vi "Keithley2612b_NOT_Measurement_DC_Supply.vi"() -> ()   [LabVIEW 2016]
uses:
  <instrlib>/Keithley 2600 Series/Public/Channel.ctl
  <instrlib>/Keithley 2600 Series/Keithley 2600 Series.lvlib
  <instrlib>/BK Precision 913XX/BK Precision 913XX.lvlib
panel:
  in  "Appand to Exist File":bool
  in  "Write to Text File?":bool
  out "Actual Current Level (A)":dbl format="%.4g"
  out "Actual Power Level (W)":dbl format="%.4g"
  out "Actual Voltage Level (V)":dbl format="%.4g"
  out "XY Graph":cluster{"Y":dbl[], "Y":dbl[]}[](graph)=[{"Y"=[-10000.0, -9899.89, -9800.119999999999, -9699.970000000001, -9600.15, -9499.96, -9400.17, -9300.01, -9199.87, -9100.09, -8999.9, -8900.119999999999, -8800.0, -8700.18, -8600.02, -8499.88, -8400.080000000002, -8299.9, -8200.1, -8099.99, -8000.159999999999, -7899.9800000000005, -7799.92, -7700.11, -7599.95, -7500.15, -7400.0599999999995, -7300.21, -7200.05, -7099.96, -7000.14, -6900.0, -6800.21, -6700.08, -6599.910000000001, -6500.17, -6400.01, -6300.169999999999, -6200.0599999999995, -6100.25, -6000.110000000001, -5899.95, -5800.18, -5700.0599999999995, -5600.21, -5500.09, -5400.25, -5300.06, -5199.97, -5100.150000000001, -5000.0, -4900.2, -4800.03, -4700.21, -4600.06, -4499.93, -4400.13, -4299.98, -4200.160000000001, -4100.04, -4000.21, -3900.1299999999997, -3799.98, -3700.13, -3599.9900000000002, -3500.1600000000003, -3399.99, -3299.84, -3200.04, -3099.88, -3000.0499999999997, -2899.9, -2800.11, -2699.9300000000003, -2599.83, -2500.0, -2399.79, -2299.98, -2199.86, -2099.9900000000002, -1999.97, -1899.98, -1799.99, -1700.0, -1600.01, -1500.01, -1400.01, -1300.0100000000002, -1200.01, -1099.99, -999.993, -900.0, -800.006, -700.009, -600.01, -500.01399999999995, -400.01300000000003, -300.0, -199.989, -99.99470000000001, 0.00660419, 100.003, 200.002, 299.978, 399.99899999999997, 500.006, 600.0060000000001, 699.975, 799.9770000000001, 899.982, 999.977, 1099.98, 1199.9899999999998, 1300.0100000000002, 1399.97, 1499.98, 1599.99, 1699.9899999999998, 1799.98, 1899.97, 1999.96, 2099.75, 2199.91, 2299.77, 2399.88, 2499.76, 2599.9, 2699.71, 2799.88, 2900.04, 2999.85, 3100.04, 3199.84, 3300.02, 3399.81, 3500.0499999999997, 3599.8, 3699.9399999999996, 3800.11, 3899.96, 4000.0400000000004, 4099.95, 4200.0599999999995, 4299.87, 4400.070000000001, 4499.889999999999, 4600.030000000001, 4699.89, 4800.049999999999, 4900.1900000000005, 5000.0, 5100.150000000001, 5200.02, 5300.099999999999, 5399.969999999999, 5500.06, 5599.88, 5700.05, 5800.19, 5900.0, 6000.12, 6099.96, 6200.08, 6299.89, 6400.04, 6499.87, 6599.95, 6700.13, 6799.92, 6900.070000000001, 6999.91, 7099.99, 7199.82, 7299.9400000000005, 7399.82, 7499.94, 7600.1, 7699.92, 7800.07, 7899.84, 8000.04, 8099.84, 8199.91, 8299.810000000001, 8399.88, 8500.0, 8599.82, 8699.970000000001, 8799.73, 8899.88, 8999.75, 9099.949999999999, 9199.72, 9299.89, 9399.73, 9499.86, 9600.03, 9699.859999999999, 9800.01, 9899.84, 10000.0], "Y"=[4939.26, 4997.93, 4998.56, 4998.95, 4999.16, 4999.38, 4999.49, 4999.64, 4999.64, 4999.780000000001, 4999.83, 4999.87, 4999.88, 4999.95, 4999.92, 5000.0, 4999.98, 5000.02, 5000.05, 5000.06, 5000.09, 5000.09, 5000.08, 5000.13, 5000.15, 5000.15, 5000.200000000001, 5000.14, 5000.200000000001, 5000.17, 5000.2300000000005, 5000.200000000001, 5000.25, 5000.2300000000005, 5000.28, 5000.24, 5000.219999999999, 5000.27, 5000.27, 5000.19, 5000.27, 5000.21, 5000.29, 5000.25, 5000.27, 5000.28, 5000.29, 5000.27, 5000.3, 5000.25, 5000.339999999999, 5000.3099999999995, 5000.3, 5000.27, 5000.3, 5000.25, 5000.3099999999995, 5000.320000000001, 5000.3099999999995, 5000.3099999999995, 5000.3, 5000.320000000001, 5000.35, 5000.33, 5000.320000000001, 5000.33, 5000.3099999999995, 5000.320000000001, 5000.29, 5000.3099999999995, 5000.320000000001, 5000.33, 5000.35, 5000.339999999999, 5000.35, 5000.36, 5000.320000000001, 5000.36, 5000.35, 5000.35, 5000.35, 5000.36, 5000.320000000001, 5000.36, 5000.35, 5000.33, 5000.339999999999, 5000.320000000001, 5000.339999999999, 5000.33, 5000.339999999999, 5000.339999999999, 5000.36, 5000.339999999999, 5000.38, 5000.35, 5000.37, 5000.35, 5000.46, 5000.339999999999, 5000.41, 5000.36, 5000.39, 5000.37, 5000.429999999999, 5000.41, 5000.4, 5000.35, 5000.42, 5000.38, 5000.42, 5000.4400000000005, 5000.41, 5000.37, 5000.38, 5000.37, 5000.320000000001, 5000.38, 5000.39, 5000.39, 5000.38, 5000.42, 5000.37, 5000.4400000000005, 5000.36, 5000.37, 5000.41, 5000.39, 5000.41, 5000.42, 5000.37, 5000.39, 5000.36, 5000.4, 5000.41, 5000.42, 5000.339999999999, 5000.41, 5000.38, 5000.45, 5000.37, 5000.45, 5000.39, 5000.41, 5000.4, 5000.429999999999, 5000.38, 5000.42, 5000.38, 5000.4, 5000.41, 5000.42, 5000.42, 5000.37, 5000.4400000000005, 5000.39, 5000.429999999999, 5000.41, 5000.41, 5000.39, 5000.45, 5000.41, 5000.46, 5000.4, 5000.41, 5000.39, 5000.4400000000005, 5000.4, 5000.48, 5000.39, 5000.4, 5000.38, 5000.429999999999, 5000.45, 5000.4, 5000.41, 5000.4, 5000.42, 5000.42, 5000.429999999999, 5000.39, 5000.4400000000005, 5000.41, 5000.42, 5000.4, 5000.4400000000005, 5000.38, 5000.42, 5000.41, 5000.45, 5000.429999999999, 5000.48, 5000.49, 5000.47, 5000.5, 5000.429999999999, 5000.47, 5000.48, 5000.49, 5000.46, 5000.46]}]
  in  "Voltage Limit (36.000 V)":dbl=36.0 min=0.0 max=66.0 step=0.001 format="%.3g"
  in  "Enable OVP (T: Enable)":bool=TRUE
  in  "Channel (1:1)":u16(ring)=1 items=["1"=1, "2"=2, "3"=3]
  in  "Current Limit (0.0 A)":dbl=1.0 min=0.0 max=25.0 step=1.0 format="%.3f"
  in  "Voltage Level (0.0 V)":dbl=5.0 format="%.3g"
  in  "DC  VISA resource name":refnum<visa-resource-name>="bk_Precision_DC_Power"
  in  "Current Limit":dbl=1.0
  out "error out":errorcluster
  in  "DC Supply Delay (s)":dbl
  in  "Start Voltage 2":dbl=-10.0
  in  "Step Size":dbl=0.1
  in  "End Voltage":dbl=10.0
  in  "Delay (s)":dbl
  in  "Reverse Sweep":bool
  in  "error in (no error)":errorcluster
  in  "Keithley VISA resource name":refnum<visa-resource-name>="Keithley_2612B"
  # "DC Power Supply Control"
  # "Input Voltage Control"
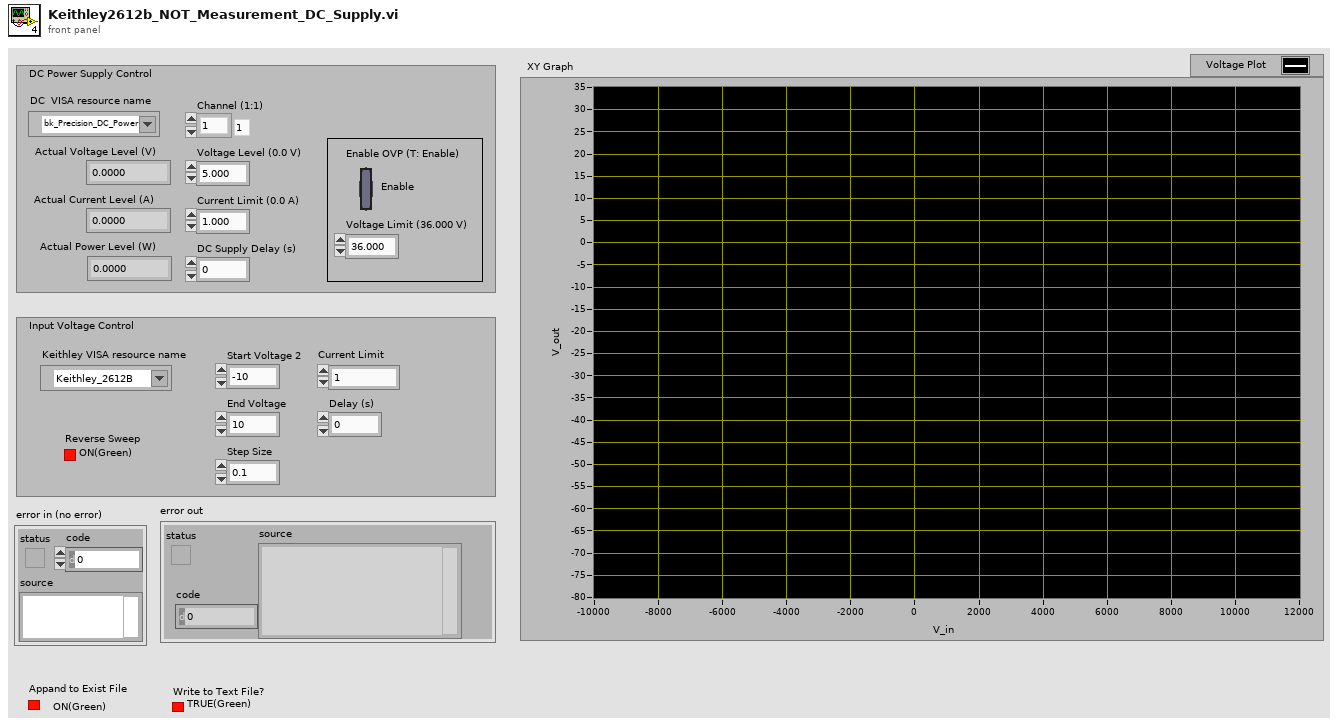
[diagram p1: front panel]
types:
  T1 = typedef "Keithley 2600 Series.lvlib/Channel.ctl" = enum32{"Channel A", "Channel B"}
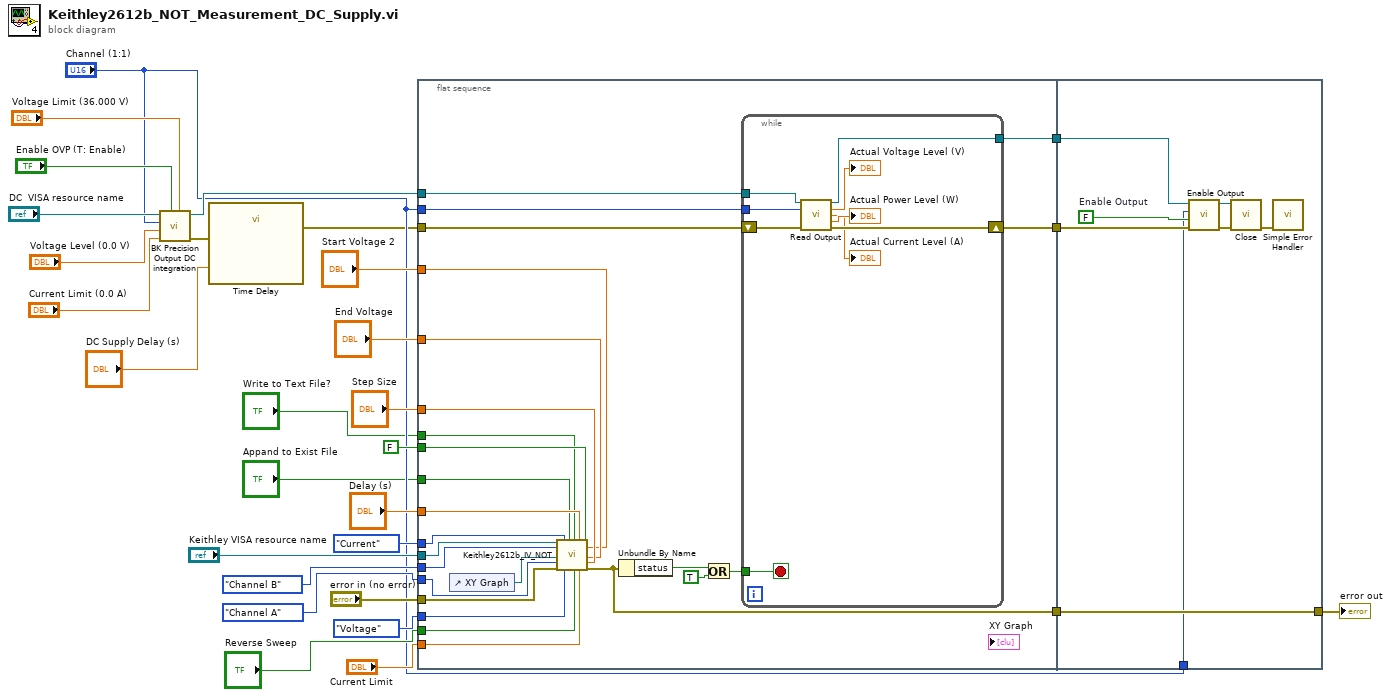
[diagram p0: block diagram]
diagram:
  n1 = call "BK Precision Output DC integration.vi"("Voltage Limit (36.000 V)"="Voltage Limit (36.000 V)", "Enable OVP (T: Enable)"="Enable OVP (T: Enable)", "Current Limit (0.0 A)"="Current Limit (0.0 A)", "Voltage Level (0.0 V)"="Voltage Level (0.0 V)", "Channel (1:1)"="Channel (1:1)", "VISA resource name"="DC  VISA resource name") -> ("error out"=w3:errorcluster, "VISA resource name out"=w7:refnum<visa-resource-name>)  [unwired: 2 in]
  n2 = call "Time Delay"("error in (no error)"=w3, "Delay Time (s)"="DC Supply Delay (s)") -> ("error out"=w4:errorcluster)  [unwired: 9 in]
  n3 = flat-sequence {
    tunnel: [w33] -> w15
    tunnel: "Current Limit" -> [w42]
    tunnel: "Start Voltage 2" -> [w43]
    tunnel: "Delay (s)" -> [w44]
    tunnel: "End Voltage" -> [w45]
    tunnel: "Step Size" -> [w46]
    tunnel: "Reverse Sweep" -> [w47]
    tunnel: enum32{"Current", "Voltage"}."Current" ("Source Function (Current)") -> [w48]
    tunnel: enum32{"Current", "Voltage"}."Voltage" ("Source Function (Current) 2") -> [w49]
    tunnel: Channel."Channel B" ("Channel (Channel A) 2") -> [w50]
    tunnel: Channel."Channel A" ("Channel (Channel A)") -> [w51]
    tunnel: "error in (no error)" -> [w52]
    tunnel: FALSE ("Error Query (False)") -> [w53]
    tunnel: "Keithley VISA resource name" -> [w54]
    tunnel: [w40] -> w8
    tunnel: w7 -> [w38]
    tunnel: [w39] -> w6
    tunnel: "Channel (1:1)" -> [w37]
    tunnel: w4 -> [w36]
    tunnel: "Appand to Exist File" -> [w31]
    tunnel: "Write to Text File?" -> [w30]
    tunnel: [w71] -> w17
    tunnel: w15 -> [w71]
    tunnel: w8 -> [w66]
    tunnel: "Channel (1:1)" -> [w64]
    tunnel: w6 -> [w65]
    frame #0 {
      n4 = control-ref of="XY Graph"() -> (w41:refnum<vi>)
      n5 = call "Keithley2612b_IV_NOT.vi"("VISA resource name"=w54, "Channel (Channel A) 2"=w50, "XY Graph Ref In"=w41, "Channel (Channel A)"=w51, "error in (no error)"=w52, "Source Function (Current)"=w48, "Source Function (Current) 2"=w49, "Appand to Exist File"=w31, "Write to Text File?"=w30, "Reverse Sweep"=w47, "Delay (s) 2"=w44, "Current Limit 2"=w42, "Error Query (False)"=w53, "Start Voltage 2"=w43, "End Voltage 2"=w45, "Step Size 2"=w46) -> ("error out"=w33:errorcluster)  [unwired: 3 in]
      n6 = Unbundle By Name(w33) -> ("status"=w34:bool)
      n7 = Or(x=w34, y=TRUE ("Stop Output")) -> (x .or. y?=w32:bool)
      n8 = while {
        tunnel: [w61] -> w39
        shift-right: [w62] -> w40
        shift-left: w36 -> [w63]
        tunnel: w38 -> [w57]
        tunnel: w37 -> [w56]
        tunnel: w32 -> [w55]
        stop <- w55 stop-if-true
        n9 = call <instrlib>:"Read Output.vi"("VISA resource name"=w57, "Channel (1:Channel 1)"=w56, "error in (no error)"=w63) -> ("VISA resource name out"=w61:refnum<visa-resource-name>, "Actual Voltage Level (V)"=→"Actual Voltage Level (V)":dbl, "Actual Current Level (A)"=→"Actual Current Level (A)":dbl, "Actual Power Level (W)"=→"Actual Power Level (W)":dbl, "error out"=w62:errorcluster)  [unwired: 8 in]
      }
    }
    frame #1 {
      w67 = FALSE  # Enable Output
      n10 = call <instrlib>:"Enable Output.vi"("error in (no error)"=w66, "Enable Output (F: False)"=w67, "Channel (1:1)"=w64, "VISA resource name"=w65) -> ("error out"=w68:errorcluster, "VISA resource name out"=w69:refnum<visa-resource-name>)  [unwired: 6 in]
      n11 = call <instrlib>:"Close.vi"("error in (no error)"=w68, "VISA resource name"=w69) -> ("error out"=w70:errorcluster)  [unwired: 9 in]
      n12 = call <vilib>:"Simple Error Handler.vi"("error in (no error)"=w70) -> ()  [unwired: 4 in, 5 out]
    }
  }
  "error out" <- w17
